vi "SQLite DB Path.vi"(11 "database":string="database1.db") -> (3 "appended path":path)   [LabVIEW 2016, in "数据查询.lvlib"]
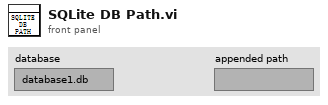
[diagram p1: front panel]
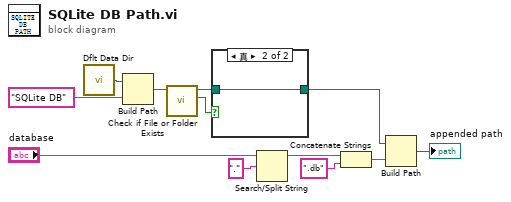
[diagram p0: block diagram]
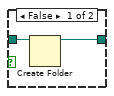
[diagram p2: hidden frame]
diagram:
  n1 = call <vilib>:"Dflt Data Dir.vi"() -> ("App:Default Data Directory"=w12:path)
  n2 = Build Path(base path=w12, name or relative path="SQLite DB" ("名称或相对路径")) -> (appended path=w9:path)
  n3 = call <vilib>:"Check if File or Folder Exists.vi"("path"=w9) -> ("file or folder exists?"=w8:bool, "dup path"=w7:path)  [unwired: 8 in, 1 out]
  n4 = case shown="真" w8 {
    tunnel: w7 -> [w14 w15]
    tunnel: [w13 w15] -> w6
    frame False {
      n5 = Create Folder(path (use dialog)=w14) -> (created path=w13:path)  [unwired: 2 in, 2 out]
    }
    frame True {
    }
  }
  n6 = Search/Split String(string="database", search string/char (-)="." ("搜索字符串/字符(-)")) -> (substring before match=w3:string)  [unwired: 1 in, 2 out]
  n7 = Concatenate Strings(w3, ".db" ("字符串")) -> (w2:string)
  n8 = Build Path(base path=w6, name or relative path=w2) -> (appended path=→"appended path":path)
